vi "Parse Message.vi"(8 "error in (no error)":errorcluster, 10 "NMEA Message":string, 11 "nmea in":refnum<class "nmea.lvclass">) -> (0 "error out":errorcluster, 3 "nmea out":refnum<class "nmea.lvclass">)   [LabVIEW 2012, in "nmea.lvlib" / "nmea.lvclass"]
uses:
  nmea.lvclass
  message/NMEA Message.lvclass
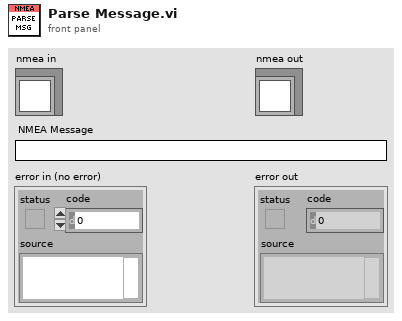
[diagram p1: front panel]
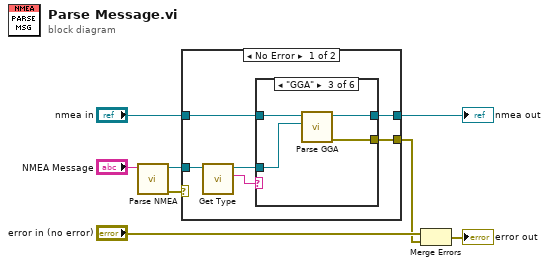
[diagram p0: block diagram]
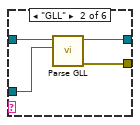
[diagram p3: hidden frame]
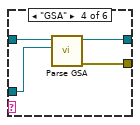
[diagram p4: hidden frame]
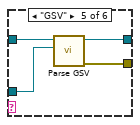
[diagram p5: hidden frame]
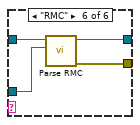
[diagram p6: hidden frame]
diagram:
  n1 = call "Parse NMEA.vi"("NMEA Line"="NMEA Message") -> ("error out"=w6:errorcluster, "NMEA Message out"=w5:refnum<class "NMEA Message.lvclass">)  [unwired: 9 in]
  n2 = case shown="No Error" w6 {
    selector: w6 -> [_ w36]
    tunnel: w5 -> [w14 _]
    tunnel: "nmea in" -> [w11 w37]
    tunnel: [w10 w37] -> w3
    tunnel: [w9 w36] -> w1
    frame No Error {
      n3 = call "Get Type.vi"("NMEA Message in"=w14) -> ("Type"=w13:string, "NMEA Message out"=w12:refnum<class "NMEA Message.lvclass">)  [unwired: 8 in, 1 out]
      n4 = case shown="\"GGA\"" w13 {
        tunnel: w12 -> [_ w16 w20 w24 w29 w34]
        tunnel: w11 -> [w15 w19 w23 w27 w31 w35]
        tunnel: [w15 w18 w22 w26 w30 w33] -> w10
        tunnel: [_ w17 w21 w25 w28 w32] -> w9
        frame Default {
        }
        frame "GLL" {
          n5 = call "Parse GLL.vi"("Message"=w16, "nmea in"=w19) -> ("error out"=w17:errorcluster, "nmea out"=w18:refnum<class "nmea.lvclass">)  [unwired: 8 in]
        }
        frame "GGA" {
          n6 = call "Parse GGA.vi"("Message"=w20, "nmea in"=w23) -> ("error out"=w21:errorcluster, "nmea out"=w22:refnum<class "nmea.lvclass">)  [unwired: 8 in]
        }
        frame "GSA" {
          n7 = call "Parse GSA.vi"("Message"=w24, "nmea in"=w27) -> ("error out"=w25:errorcluster, "nmea out"=w26:refnum<class "nmea.lvclass">)  [unwired: 8 in]
        }
        frame "GSV" {
          n8 = call "Parse GSV.vi"("Message"=w29, "nmea in"=w31) -> ("error out"=w28:errorcluster, "nmea out"=w30:refnum<class "nmea.lvclass">)  [unwired: 8 in]
        }
        frame "RMC" {
          n9 = call "Parse RMC.vi"("Message"=w34, "nmea in"=w35) -> ("error out"=w32:errorcluster, "nmea out"=w33:refnum<class "nmea.lvclass">)  [unwired: 8 in]
        }
      }
    }
    frame Error {
    }
  }
  "nmea out" <- w3
  n10 = Merge Errors("error in (no error)", w1) -> (→"error out":errorcluster)
